vi "test_Feature Tracking_distance.vi"() -> ()   [LabVIEW 2020]
doc: "This example shows how to use the Lucas Kanade Pyramid motion estimation VI to track features in a sequence of images in NI Vision. The VI reads the frames from an AVI file and tracks user specified features in the image from frame to frame."
uses:
  <vilib>/vision/NI_Vision_Development_Module.lvlib
panel:
  out "Waveform Graph":dbl[][](graph)
  out "Array":dbl[][](array[numeric])
  out "Distance Array":dbl[](array[numeric]) caption="DistanceArray"
  in  "Delay (s.)":dbl(slide)=0.25 scale=0.0..1.5
  out "Image":T1(plugin-control)
  out "Progress Bar":i32(slide) max=29 scale=0.0..29.0
  in  "Stop":bool
  # "Overview: Demonstrate the use of the Optical Flow tracking algorithm of Vision Development Module.\nRequirements: Vision Development Module\nInstructions: Run the VI."
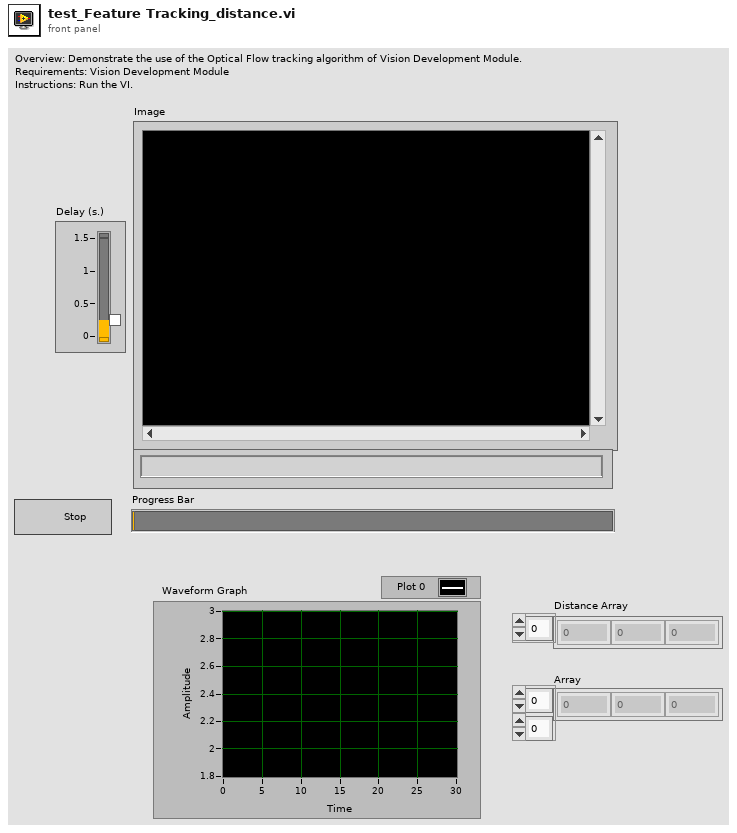
[diagram p1: front panel]
types:
  T1 = typedef "IMAQ Image.ctl" = refnum<image>
  T2 = cluster{"Particle Measurements (Pixels)[0]":dbl, "Particle Measurements (Pixels)[1]":dbl}[]
  T3 = cluster{"Level":i32, "Max. Iterations":i32, "Window Size":i32, "Displacement Threshold":dbl}
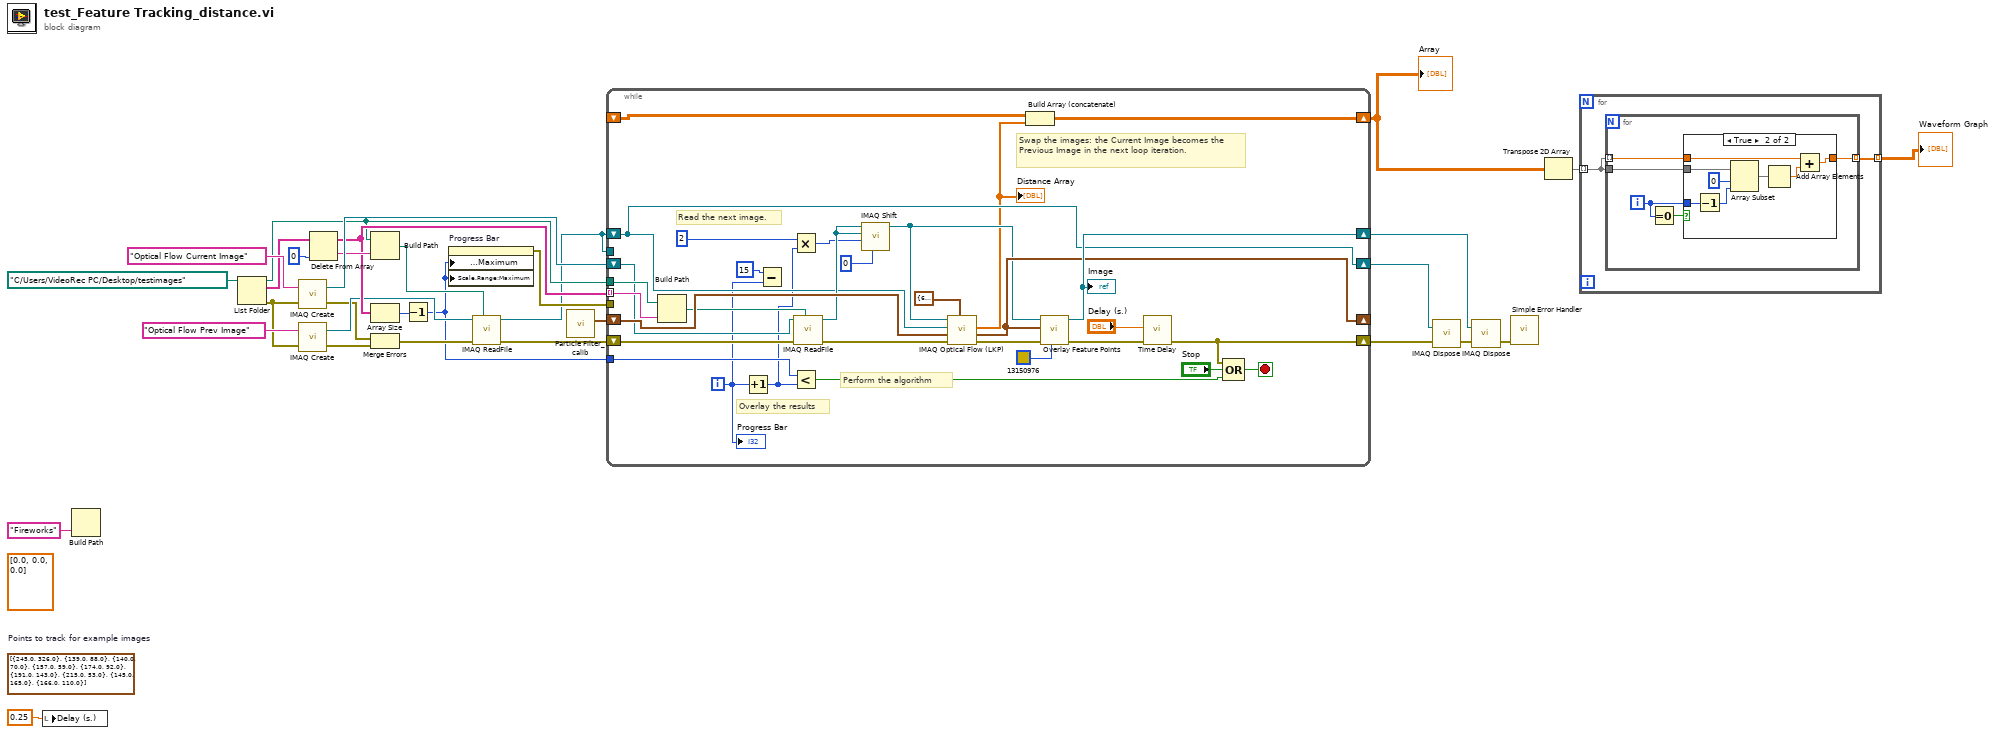
[diagram p0: block diagram]
diagram:
  (unwired) dbl[] [0.0, 0.0, 0.0]
  (unwired) cluster{"X":sgl, "Y":sgl}[] [{"X"=245.0, "Y"=326.0}, {"X"=139.0, "Y"=88.0}, {"X"=140.0, "Y"=70.0}, {"X"=157.0, "Y"=59.0}, {"X"=174.0, "Y"=92.0}, {"X"=191.0, "Y"=143.0}, {"X"=215.0, "Y"=53.0}, {"X"=145.0, "Y"=165.0}, {"X"=166.0, "Y"=110.0}]  # Points to track for example images
  n1 = local write "Delay (s.)"(0.25 ("Delay (s)")) -> ()
  n2 = Build Path(name or relative path="Fireworks") -> ()  [unwired: 1 in, 1 out]
  n3 = List Folder(path=path "C:/Users/VideoRec PC/Desktop/testimages") -> (path out=w6:path, filenames=w20:string[], error out=w16:errorcluster)  [unwired: 1 in, 3 out]
  n4 = call "IMAQ Create"("Image Name"="Optical Flow Current Image", "error in (no error)"=w16) -> ("New Image"=w30:T1, "error out"=w15:errorcluster)  [unwired: 2 in, 1 out]
  n5 = call "IMAQ Create"("Image Name"="Optical Flow Prev Image", "error in (no error)"=w16) -> ("New Image"=w21:T1, "error out"=w14:errorcluster)  [unwired: 2 in, 1 out]
  n6 = Delete From Array(array=w20, index=0) -> (deleted portion=w26:string, array with subset deleted=w24:string[])  [unwired: 1 in]
  n7 = Build Path(base path=w6, name or relative path=w26) -> (appended path=w22:path)
  n8 = Array Size(array=w24) -> (size(s)=w25:i32)
  n9 = Merge Errors(w15, w14) -> (w13:errorcluster)
  n10 = Decrement(x=w25) -> (x-1=w9:i32)
  n11 = property on="Progress Bar" class="Slide (strict)"("Data Entry Limits:Maximum"=w9, "Scale.Range:Maximum"=w9) -> (error out=w29:errorcluster)  [unwired: 2 in, 1 out]
  n12 = call "IMAQ ReadFile"("File Path"=w22, "error in (no error)"=w13, "Image"=w21) -> ("error out"=w23:errorcluster, "Image Out"=w4:T1)  [unwired: 2 in, 5 out]
  n13 = call "Particle Filter_calib.vi"() -> ("Location in Pixels"=w5:T2)  [unwired: 9 in, 2 out]
  n14 = while {
    tunnel: w9 -> [w59]
    tunnel: w29 -> [_]
    shift-right: [w58] -> w18
    shift-left: w4 -> [w39]
    shift-right: [w56] -> _
    shift-left: w5 -> [w57]
    shift-right: [w54] -> w17
    shift-left: w23 -> [w62]
    tunnel: w6 -> [w55]
    tunnel: w24 -> [w47] mode=indexing
    shift-right: [w39] -> w19
    shift-left: w30 -> [w43]
    tunnel: w4 -> [_]
    shift-right: [w34] -> w2
    shift-left: _ -> [w35]
    i -> [w36]
    stop <- w46 stop-if-true
    # "Swap the images: the Current Image becomes the Previous Image in the next loop iteration."
    # "Overlay the results"
    # "Read the next image."
    # "Perform the algorithm"
    n15 = Build Path(base path=w55, name or relative path=w47) -> (appended path=w48:path)
    n16 = Increment(x=w36) -> (x+1=w32:i32)
    n17 = Subtract(x=15, y=w36) -> ()  [unwired: 1 out]
    n18 = Multiply(x=2, y=w32) -> (x*y=w38:i32)
    n19 = Less?(x=w59, y=w32) -> (x < y?=w61:bool)
    n20 = call "IMAQ ReadFile"("File Path"=w48, "error in (no error)"=w62, "Image"=w43) -> ("error out"=w51:errorcluster, "Image Out"=w42:T1)  [unwired: 2 in, 5 out]
    n21 = call "IMAQ Shift"("YOffset"=0, "XOffset"=w38, "Image Dst"=w42, "Image Src"=w42) -> ("Image Dst Out"=w41:T1)  [unwired: 6 in, 1 out]
    n22 = call "IMAQ Optical Flow (LKP)"("Options"=T3 {"Level"=6, "Max. Iterations"=20, "Window Size"=50, "Displacement Threshold"=0.01}, "error in (no error)"=w51, "Feature Points In"=w57, "Previous Frame"=w39, "Current Frame"=w41) -> ("error out"=w50:errorcluster, "Feature Points Out"=w56:cluster{"X":sgl, "Y":sgl}[], "Distance Array"=w33:dbl[])  [unwired: 1 in, 3 out]
    "Distance Array" <- w33
    n23 = Build Array (concatenate)(w35, w33) -> (w34:dbl[][])
    n24 = call "Overlay Feature Points.vi"("Color"=u32 13150976, "error in"=w50, "Feature Points"=w56, "Image"=w41) -> ("error out"=w52:errorcluster, "Image Out"=w58:T1)  [unwired: 2 in, 4 out]
    "Image" <- w58
    n25 = call "Time Delay"("error in (no error)"=w52, "Delay Time (s)"="Delay (s.)") -> ("error out"=w54:errorcluster)  [unwired: 9 in]
    n26 = Compound Arithmetic op=OR(w54, "Stop", w61) -> (w46:bool)
    "Progress Bar" <- w36
  }
  "Array" <- w2
  n27 = call "IMAQ Dispose"("Image"=w19, "error in (no error)"=w17) -> ("error out"=w11:errorcluster)  [unwired: 1 in, 3 out]
  n28 = call "IMAQ Dispose"("Image"=w18, "error in (no error)"=w11) -> ("error out"=w10:errorcluster)  [unwired: 1 in, 3 out]
  n29 = call <vilib>:"Simple Error Handler.vi"("error in (no error)"=w10) -> ()  [unwired: 1 in, 8 out]
  n30 = Transpose 2D Array(2D array=w2) -> (transposed array=w3:dbl[][])
  n31 = for {
    tunnel: w3 -> [w64] mode=indexing
    tunnel: [w63] -> w1 mode=indexing
    n32 = for {
      tunnel: w64 -> [w69] mode=indexing
      tunnel: w64 -> [w68]
      tunnel: [w67] -> w63 mode=indexing
      i -> [w66]
      n33 = Equal To 0?(x=w66) -> (x = 0?=w65:bool)
      n34 = case shown="True" w65 {
        tunnel: w69 -> [w70 w78]
        tunnel: w66 -> [_ w77]
        tunnel: w68 -> [_ w76]
        tunnel: [w70 w74] -> w67
        frame False {
        }
        frame True {
          n35 = Decrement(x=w77) -> (x-1=w73:i32)
          n36 = Array Subset(array=w76, index=0, length=w73) -> (w75:dbl[])
          n37 = Add Array Elements(numeric array=w75) -> (sum=w71:dbl)
          n38 = Add(x=w78, y=w71) -> (x+y=w74:dbl)
        }
      }
    }
  }
  "Waveform Graph" <- w1
